vi "HQ Main.vi"() -> ()   [LabVIEW 2014]
uses:
  Type Defs/PodHealth.ctl
  Type Defs/PodStates.ctl
  Type Defs/PodState.ctl
panel:
  out "Pod States":T1
  out "Pusher Attached":bool
  in  "Phase":T2={"Pre-Flight Tests"=FALSE, "Ready"=FALSE, "Accelerate"=TRUE, "Coast"=FALSE, "Brake"=FALSE, "Post-Flight"=FALSE}
  in  "Detail Window":T3(tab)
  in  "Reset Sensors":bool
  in  "Vent":bool
  in  "Brake Boost":bool
  in  "Brake Open":bool
  in  "Sensor Power":bool
  in  "Activate Pneumatics":bool
  in  "Friction Brake":bool
  in  "Mag Brake":bool
  in  "Levitation":bool
  out "Pressure":T4(graph)
  out "Levitation Gap (mm)":T5(graph)
  out "Battery Monitor":cluster{"Voltage (Total)":dbl, "Power":dbl}(graph)={"Voltage (Total)"=11.91201, "Power"=9.516504789}
  in  "Run ToF Calibration":bool=TRUE
  in  "Send Non-Critical Data":bool=TRUE
  in  "Stop":bool
  out "Battery Current":dbl(knob)=9.144776890538314 scale=0.0..5.0
  out "Battery Voltage":dbl(knob)=11.942438656676648 scale=11.0..12.0
  out "Batt. Temp":dbl(slide)=81.63265306122449 scale=0.0..100.0
  out "Gap 4":u8(slide)=11 scale=0.0..100.0
  out "Gap 3":u8(slide)=10 scale=0.0..200.0
  out "Gap 2":u8(slide)=12 scale=0.0..100.0
  out "Gap 1":u8(slide)=13 scale=0.0..100.0
  in  "Track Position":dbl(slide)=438.0053908355795 scale=0.0..5000.0
  out "Pod Health":T6={"Overall Pod Health"=TRUE, "Power"={"Power"=TRUE, "Friction Brakes"=TRUE, "Magnetic Brakes"=TRUE, "Primary Battery"=TRUE, "Backup Battery"=TRUE}, "Pressure"={"Pressure"=TRUE, "HP"=TRUE, "MP "=TRUE, "LP"=TRUE}, "Position"={"Position"=TRUE, "Maglock"=TRUE, "Levitation (ToF)"=TRUE}}
  # "TBD kick off calibration on ToF"
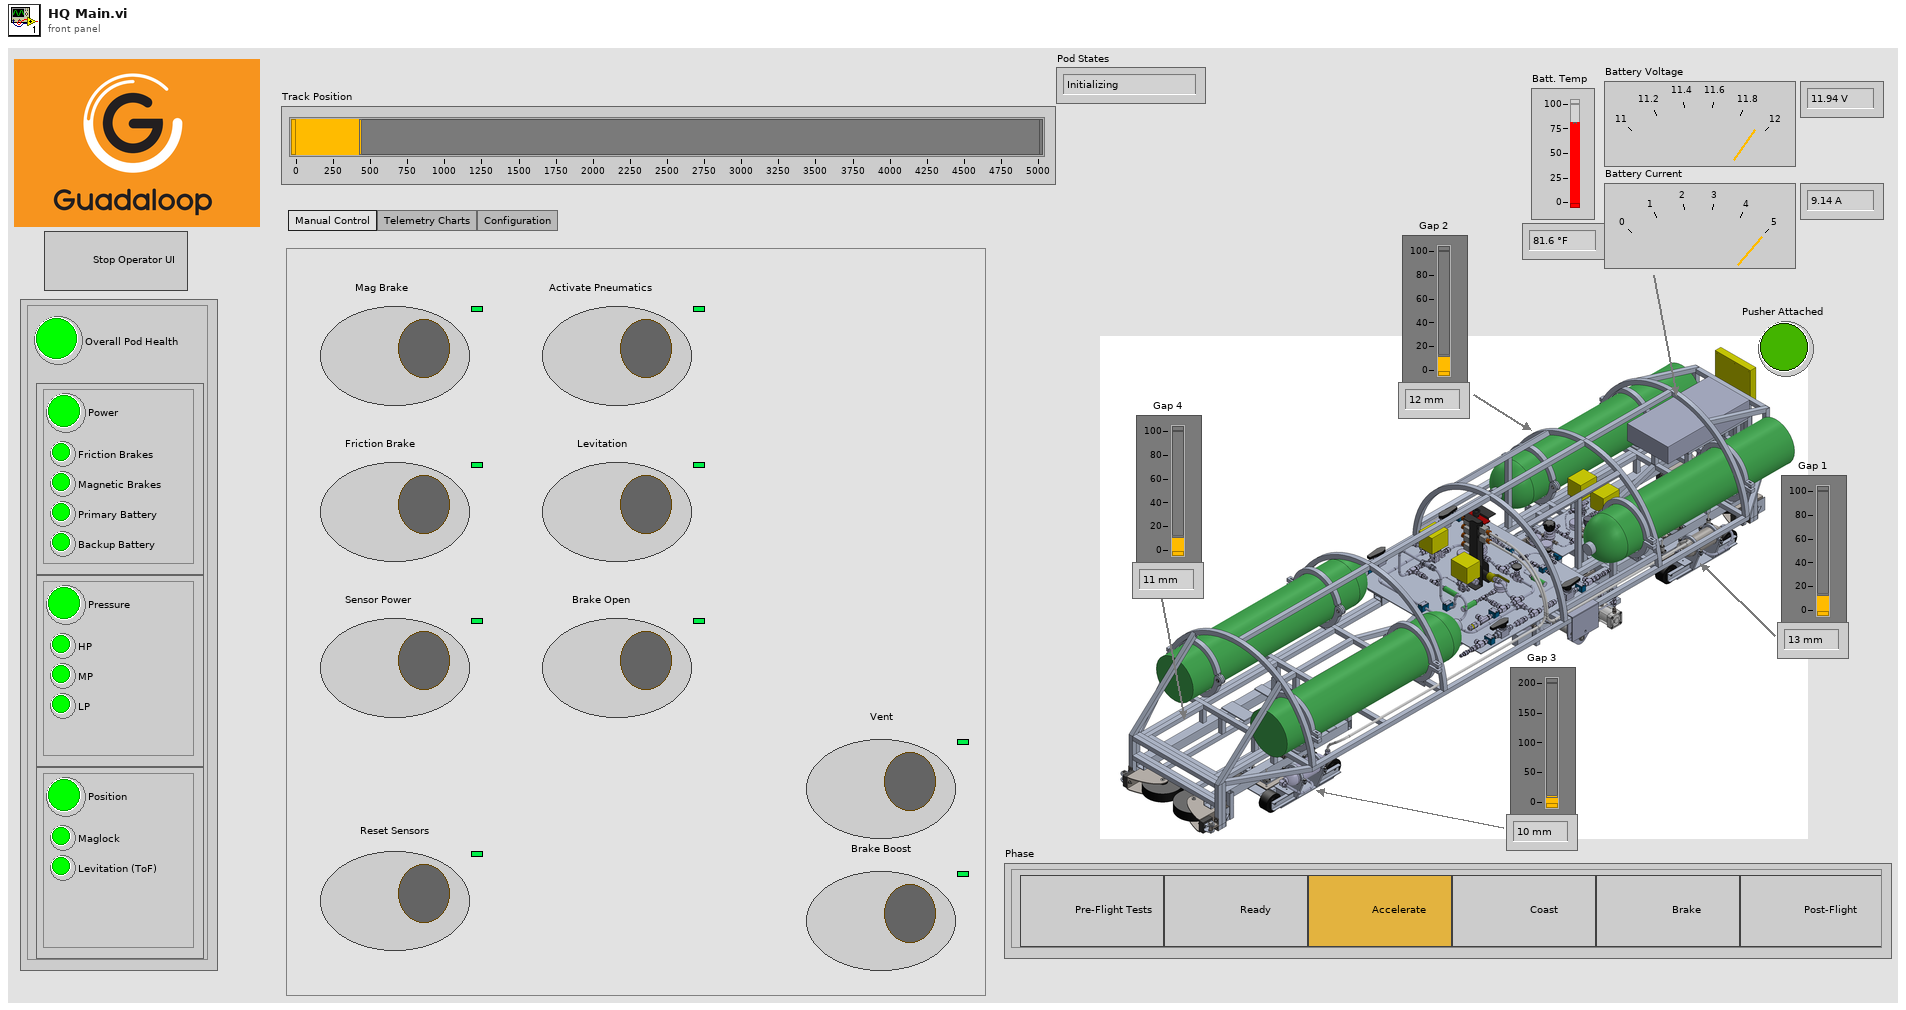
[diagram p1: front panel]
types:
  T1 = typedef "PodState.ctl" = enum16{"Initializing", "Pre-flight Testing", "Ready", "Pushing", "Coast", "Braking", "Post-flight", "Fault"}
  T2 = typedef "PodStates.ctl" = cluster{"Pre-Flight Tests":bool, "Ready":bool, "Accelerate":bool, "Coast":bool, "Brake":bool, "Post-Flight":bool}
  T3 = enum32{"Manual Control", "Telemetry Charts", "Configuration"}
  T4 = cluster{"Double":dbl, "Double":dbl, "Double":dbl, "Double":dbl}
  T5 = cluster{"UInt8":u8, "UInt8":u8, "UInt8":u8, "UInt8":u8}
  T6 = typedef "PodHealth.ctl" = cluster{"Overall Pod Health":bool, "Power":cluster{"Power":bool, "Friction Brakes":bool, "Magnetic Brakes":bool, "Primary Battery":bool, "Backup Battery":bool}, "Pressure":cluster{"Pressure":bool, "HP":bool, "MP ":bool, "LP":bool}, "Position":cluster{"Position":bool, "Maglock":bool, "Levitation (ToF)":bool}}
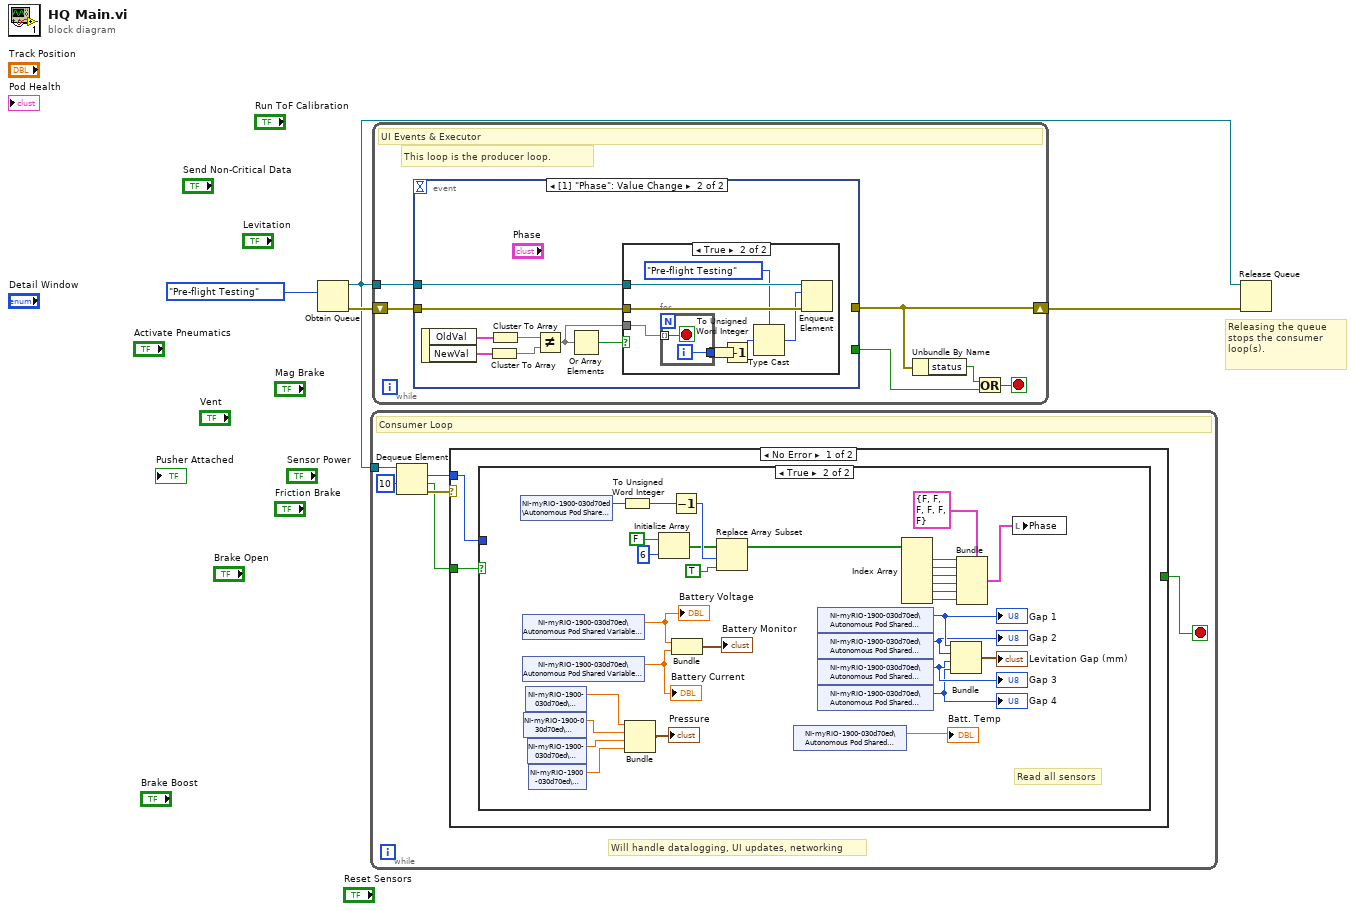
[diagram p0: block diagram]
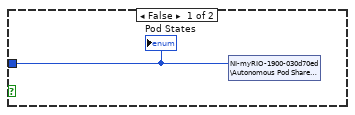
[diagram p2: hidden frame]
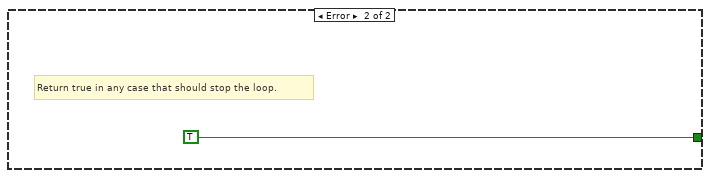
[diagram p3: hidden frame]
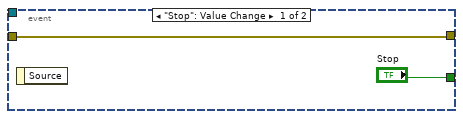
[diagram p4: hidden frame]
diagram:
  # "Releasing the queue stops the consumer loop(s)."
  n1 = Obtain Queue(element data type=PodState."Pre-flight Testing" ("Pod States")) -> (queue out=w2:refnum<queue>, error out=w4:errorcluster)  [unwired: 4 in, 1 out]
  n2 = while {
    tunnel: w2 -> [w10]
    stop <- w7 stop-if-true
    # "Will handle datalogging, UI updates, networking"
    # "Consumer Loop"
    n3 = Dequeue Element(queue=w10, timeout in ms (-1)=10) -> (element=w8:T1, timed out?=w5:bool, error out=w9:errorcluster)  [unwired: 1 in, 1 out]
    n4 = case shown="No Error" w9 {
      tunnel: w8 -> [w11 _]
      tunnel: [_ TRUE] -> w7
      tunnel: w5 -> [w12 _]
      frame No Error {
        n5 = case shown="True" w12 {
          tunnel: w11 -> [w13 _]
          frame False {
            n6 = shared-variable "NI-myRIO-1900-030d70ed\\Autonomous Pod Shared Variables.lvlib\\PodState"(w13) -> ()  [unwired: 1 in, 1 out]
            "Pod States" <- w13
          }
          frame True {
            # "Read all sensors"
            n7 = shared-variable "NI-myRIO-1900-030d70ed\\Autonomous Pod Shared Variables.lvlib\\PodState"() -> (w43:T1)  [unwired: 1 in, 1 out]
            n8 = shared-variable "NI-myRIO-1900-030d70ed\\Autonomous Pod Shared Variables.lvlib\\BatteryVoltage"() -> (w19:dbl)  [unwired: 1 in, 1 out]
            "Battery Voltage" <- w19
            n9 = shared-variable "NI-myRIO-1900-030d70ed\\Autonomous Pod Shared Variables.lvlib\\BatteryCurrent"() -> (w18:dbl)  [unwired: 1 in, 1 out]
            "Battery Current" <- w18
            n10 = shared-variable "NI-myRIO-1900-030d70ed\\Autonomous Pod Shared Variables.lvlib\\MP"() -> (w25:dbl)  [unwired: 1 in, 1 out]
            n11 = shared-variable "NI-myRIO-1900-030d70ed\\Autonomous Pod Shared Variables.lvlib\\HP"() -> (w26:dbl)  [unwired: 1 in, 1 out]
            n12 = shared-variable "NI-myRIO-1900-030d70ed\\Autonomous Pod Shared Variables.lvlib\\BP"() -> (w24:dbl)  [unwired: 1 in, 1 out]
            n13 = shared-variable "NI-myRIO-1900-030d70ed\\Autonomous Pod Shared Variables.lvlib\\LP"() -> (w23:dbl)  [unwired: 1 in, 1 out]
            n14 = To Unsigned Word Integer(number=w43) -> (unsigned 16bit integer=w29:u16)
            n15 = Bundle("Double"=w26, "Double"=w25, "Double"=w24, "Double"=w23) -> (→"Pressure":T4)  [unwired: 1 in]
            n16 = Initialize Array(FALSE, 6 ("dimension size")) -> (w32:bool[])
            n17 = Decrement(x=w29) -> (x-1=w34:u16)
            n18 = Bundle("Double"=w19, "Double"=w18) -> (→"Battery Monitor":cluster{"Double":dbl, "Double":dbl})  [unwired: 1 in]
            n19 = Replace Array Subset(array=w32, new element=TRUE, index=w34) -> (w36:bool[])
            n20 = shared-variable "NI-myRIO-1900-030d70ed\\Autonomous Pod Shared Variables.lvlib\\BatteryTemp"() -> (→"Batt. Temp":dbl)  [unwired: 1 in, 1 out]
            n21 = shared-variable "NI-myRIO-1900-030d70ed\\Autonomous Pod Shared Variables.lvlib\\ToF1Distance"() -> (w17:u8)  [unwired: 1 in, 1 out]
            "Gap 1" <- w17
            n22 = shared-variable "NI-myRIO-1900-030d70ed\\Autonomous Pod Shared Variables.lvlib\\ToF2Distance"() -> (w16:u8)  [unwired: 1 in, 1 out]
            "Gap 2" <- w16
            n23 = shared-variable "NI-myRIO-1900-030d70ed\\Autonomous Pod Shared Variables.lvlib\\ToF3Distance"() -> (w15:u8)  [unwired: 1 in, 1 out]
            "Gap 3" <- w15
            n24 = shared-variable "NI-myRIO-1900-030d70ed\\Autonomous Pod Shared Variables.lvlib\\ToF4Distance"() -> (w14:u8)  [unwired: 1 in, 1 out]
            "Gap 4" <- w14
            n25 = Index Array(array=w36) -> (element #1=w37:bool, element #2=w38:bool, element #3=w39:bool, element #4=w40:bool, element #5=w41:bool, element #6=w42:bool)  [unwired: 6 in]
            n26 = Bundle("UInt8"=w17, "UInt8"=w16, "UInt8"=w15, "UInt8"=w14) -> (→"Levitation Gap (mm)":T5)  [unwired: 1 in]
            n27 = Bundle(cluster=T2 {"Pre-Flight Tests"=FALSE, "Ready"=FALSE, "Accelerate"=FALSE, "Coast"=FALSE, "Brake"=FALSE, "Post-Flight"=FALSE} ("Phase"), "Pre-Flight Tests"=w37, "Ready"=w38, "Accelerate"=w39, "Coast"=w40, "Brake"=w41, "Post-Flight"=w42) -> (w28:T2)
            n28 = local write "Phase"(w28) -> ()
          }
        }
      }
      frame Error {
        # "Return true in any case that should stop the loop."
      }
    }
  }
  n29 = while {
    shift-right: [w46] -> w3
    shift-left: w4 -> [w49]
    tunnel: w2 -> [w50]
    stop <- w47 stop-if-true
    # "This loop is the producer loop."
    # "UI Events & Executor"
    n30 = event shown="[1] \"Phase\": Value Change" {
      selector: _ -> [_ _]
      dyn-events: _ -> [_ _]
      timeout: _ -> [_ _]
      tunnel: w50 -> [_ w59]
      tunnel: w49 -> [w52 w58]
      tunnel: [w52 _] -> w46
      tunnel: ["Stop" _] -> w48
      event "Stop": Value Change {
        n31 = event-data() -> ()  [unwired: 1 in, 1 out]
      }
      event Value Change {
        n32 = event-data() -> ("OldVal"=w60:T2, "NewVal"=w57:T2)  [unwired: 1 in]
        n33 = Cluster To Array(cluster=w57) -> (array=w55:bool[])
        n34 = Cluster To Array(cluster=w60) -> (array=w56:bool[])
        n35 = Not Equal?(x=w56, y=w55) -> (x != y?=w53:bool[])
        n36 = Or Array Elements(Boolean array=w53) -> (logical OR=w54:bool)
        n37 = case shown="True" w54 {
          tunnel: w59 -> [_ w68]
          tunnel: w58 -> [_ w67]
          tunnel: w53 -> [_ w66]
          frame False {
          }
          frame True {
            n38 = for {
              tunnel: w66 -> [w70] mode=indexing
              tunnel: [w69] -> w65
              i -> [w69]
              stop <- w70 stop-if-true
            }
            n39 = To Unsigned Word Integer(number=w65) -> (unsigned 16bit integer=w61:u16)
            n40 = Increment(x=w61) -> (x+1=w62:u16)
            n41 = Type Cast(type=PodState."Pre-flight Testing" ("Pod States"), x=w62) -> (*(type *) &x=w63:T1)
            n42 = Enqueue Element(queue=w68, element=w63, error in (no error)=w67) -> ()  [unwired: 1 in, 3 out]
          }
        }
      }
    }
    n43 = Unbundle By Name(w46) -> ("status"=w45:bool)
    n44 = Or(x=w45, y=w48) -> (x .or. y?=w47:bool)
  }
  n45 = Release Queue(queue=w2, error in (no error)=w3) -> ()  [unwired: 1 in, 3 out]
